vi "FormCalibra11-joao.vi"() -> ()   [LabVIEW 2014]
uses:
  testMachine.ctl
  mainMachine.ctl
  <vilib>/Instr/_visa.llb/VISA Configure Serial Port (Instr).vi
  <vilib>/express/express shared/transition.llb/Dynamic To Waveform Array.vi
  <vilib>/express/express signal manip/GetorSetDDTAttributes/Set DDT Attributes/SetT0.vi
  <vilib>/express/express shared/transition.llb/Waveform Array To Dynamic.vi
  <vilib>/express/express signal manip/GetorSetDDTAttributes/Set DDT Attributes/Set DDT Properties.xnode
panel:
  out "editVibration":dbl caption="Vibration (mg)" format="%#_4f"
  in  "editOffsetForce 3":dbl caption="Tare (Kgf)" min=-100.0 max=100.0 step=0.1
  out "editForce 3":dbl caption="Force (Kgf)" format="%#_4f"
  in  "editOffsetForce 2":dbl caption="Tare (Kgf)" min=-100.0 max=100.0 step=0.1
  out "editForce 2":dbl caption="Force (Kgf)" format="%#_4f"
  in  "editSetTempRefB":dbl caption="Offset B" step=0.01 format="%#_2f"
  in  "VISA Serial Port":refnum<visa-resource-name>
  in  "Lower level":dbl
  in  "hysteresis":dbl format="%.2p"
  in  "level":dbl format="%.2p"
  out "rpm":bool
  out "editTotalWaitLimit":u8
  out "editCountWaitLimit":u8
  out "ledWaitState":bool caption="Wait State"
  out "sliderWaitUpperTime":u8(slide) max=50 scale=0.0..30.0
  out "slideWaitLowerTime":u8(slide) max=30 scale=0.0..1.0
  out "slideWaitTime":u8(slide) scale=0.0..50.0
  out "labelTestTime":string caption="Tempo total de ensaio"
  in  "editSetWaitTime":u8 caption="Interval between snubs (s)" step=1 format="%0d"
  in  "stop":bool
  out "ledAcquireState":bool caption="Acquire State"
  out "editTotalLowerLimit":u8
  out "editCountLowerLimit":u8
  out "editTotalUpperLimit":u8
  out "editCountUpperLimit":u8
  out "ledEnsaio 3":bool
  out "ledBrakeState":bool caption="Brake State"
  out "ledExitState":bool caption="Exit State"
  out "ledMotorState":bool caption="Motor State"
  out "ledInit2State":bool caption="Init State"
  out "ledBlockState":bool caption="Block State"
  out "ledRunningState":bool caption="Running State"
  out "ledReadyState":bool caption="Ready State"
  out "ledInitState":bool caption="Init State"
  out "mainMachine":T1
  out "testMachine":T2=enum."finish"
  in  "editSetPathToFile":path
  in  "buttonStop":bool
  in  "buttonStart":bool
  in  "editOffsetForce":dbl caption="Tare (Kgf)" min=-100.0 max=100.0 step=0.1
  out "editForce":dbl caption="Force (Kgf)" format="%#_4f"
  out "editRPM":dbl caption="RPM" format="%#_4f"
  out "editFrequency":dbl caption="Frequency (Hz)" format="%#_4f"
  in  "editSetWaitLowerTime":u8 caption="Lower Wait Interval (s)"
  in  "editSetWaitUpperTime":u8=3 caption="Upper Wait Interval (s)"
  in  "editSetNumberOfCycles":u16 caption="Number of snubs" max=999 step=1 format="%0d"
  in  "editSetLowerLimit":u32 caption="Lower Limit (RPM)"
  in  "editSetUpperLimit":u32 caption="Upper Limit (RPM)"
  out "editTempB":dbl caption="Temperature B (ºC)"
  out "editTempA":dbl caption="Temperature A (ºC)"
  in  "editSetTempRefA":dbl caption="Offset A" step=0.01 format="%#_2f"
  out "ledMotor":bool
  out "ledBrake":bool
  out "ledEnsaio":bool
  out "labelTotalCycle":string
  out "labelCurrentCycle":string
  out "labelSystemTitle":string
  in  "editCurrCycleCtr":u32
  in  "velocidade 2":u32
  out "velocidade":u32
  # "Brake Test Bench"
  # "Com Port"
  # "Temperature"
  # "Rotation"
  # "Load Cell"
  # "Accelerometer"
  # "Test Configuration"
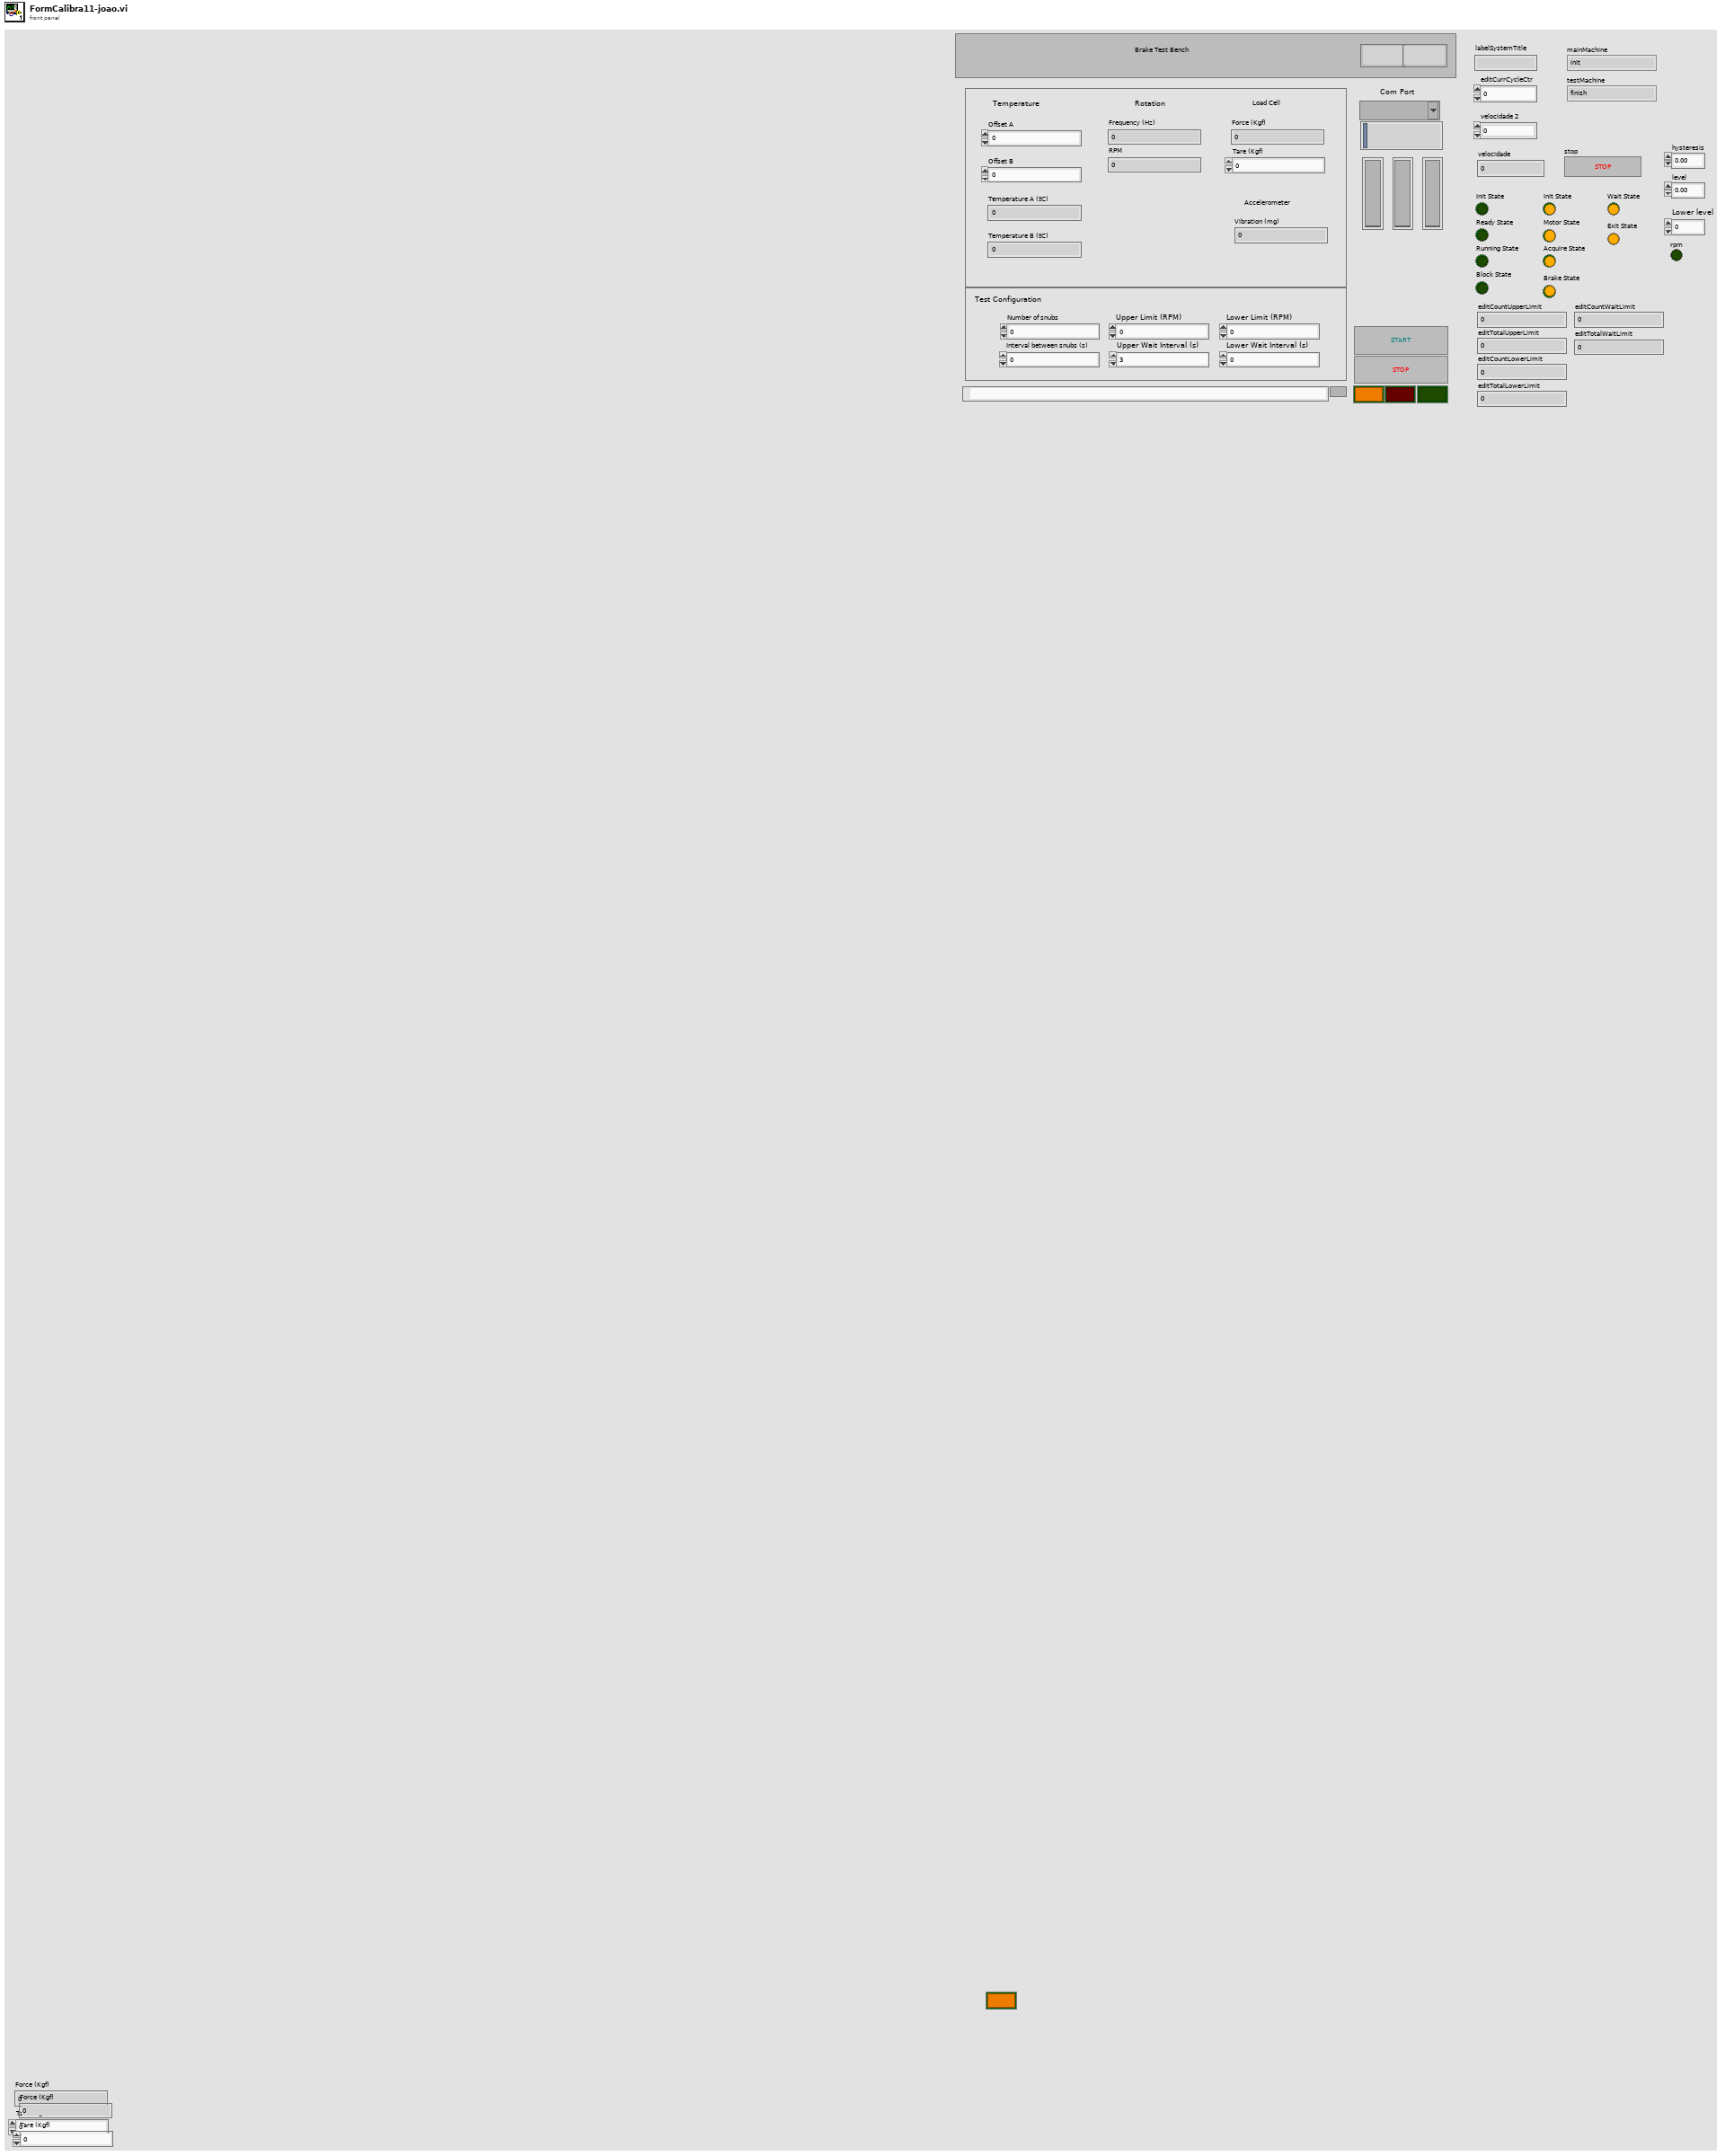
[diagram p1: front panel]
types:
  T1 = typedef "mainMachine.ctl" = enum16{"init", "ready", "running", "blocked", "finish"}
  T2 = typedef "testMachine.ctl" = enum16{"init", "motor", "motor acquire", "brake", "brake acquire", "wait ", "finish", "exit"}
  T3 = enum8{"Enabled", "Disabled", "Disabled and Grayed Out"}
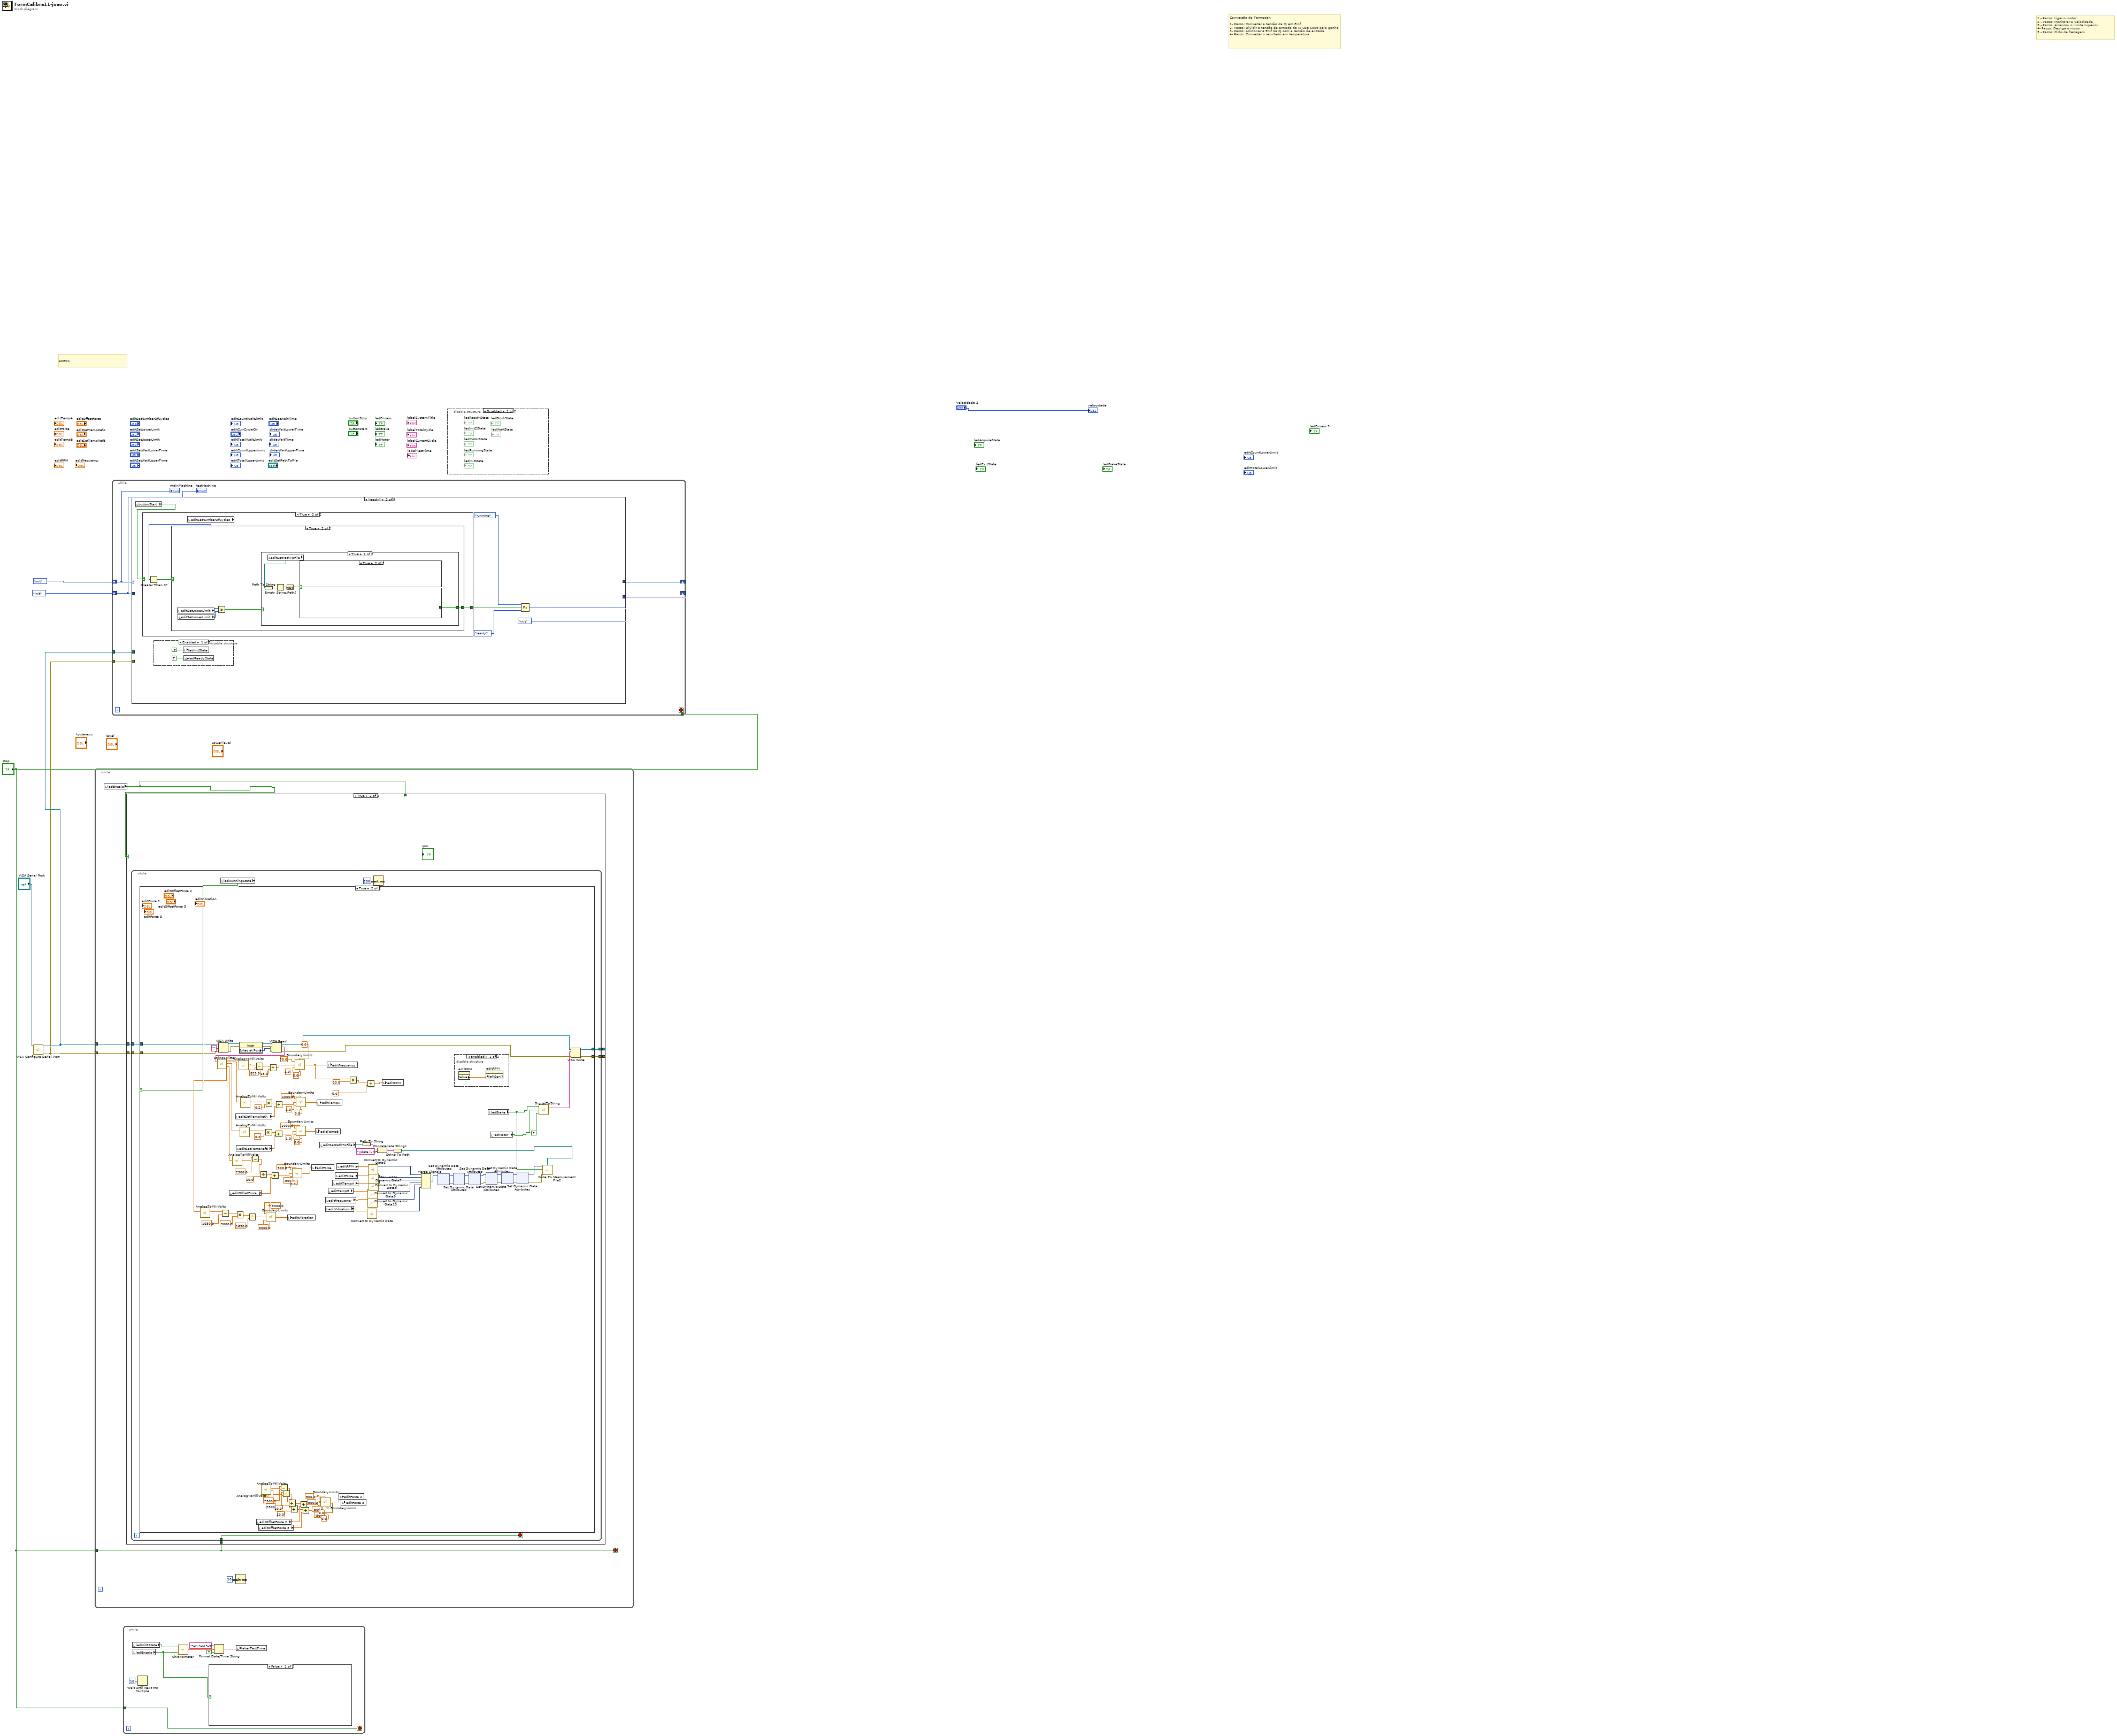
[diagram p0: block diagram]
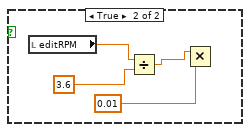
[diagram p3: hidden frame]
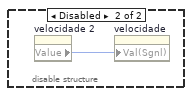
[diagram p6: hidden frame]
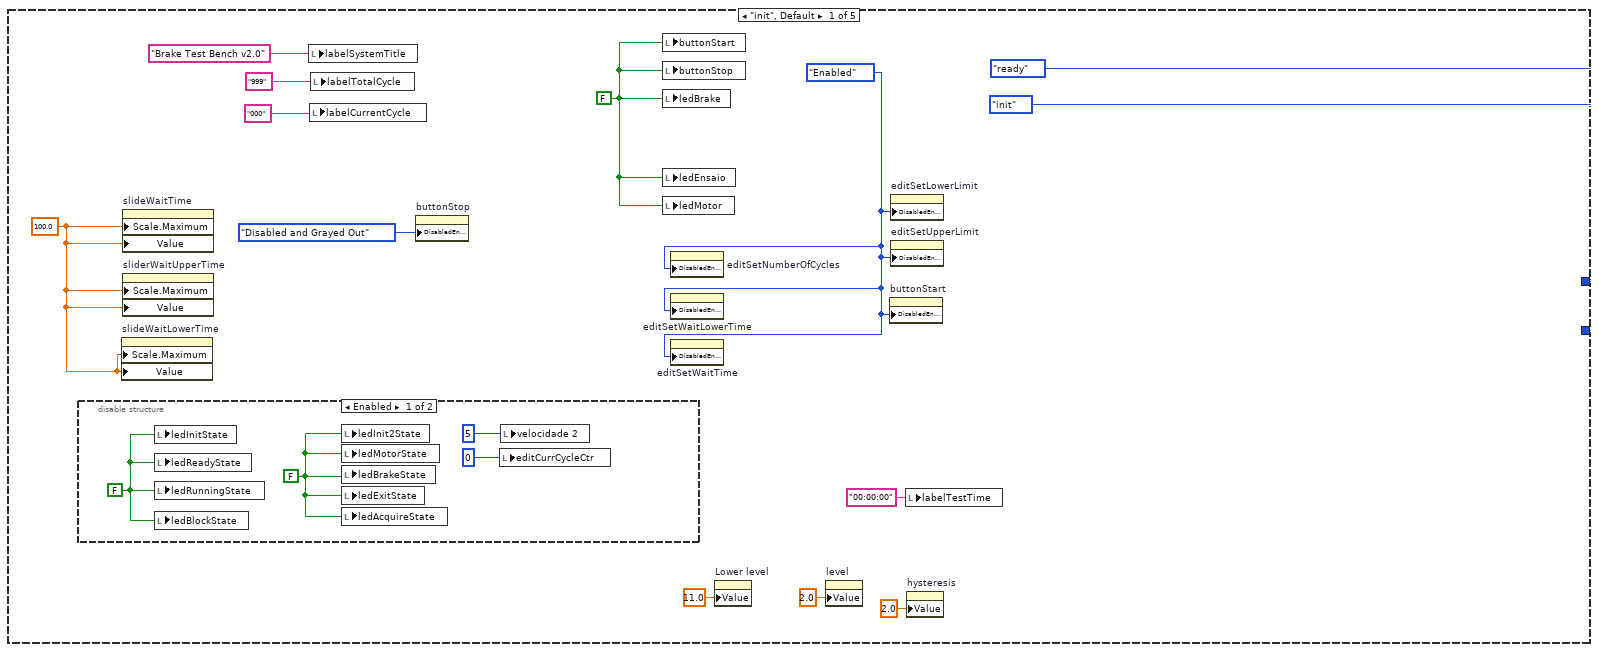
[diagram p7: hidden frame]
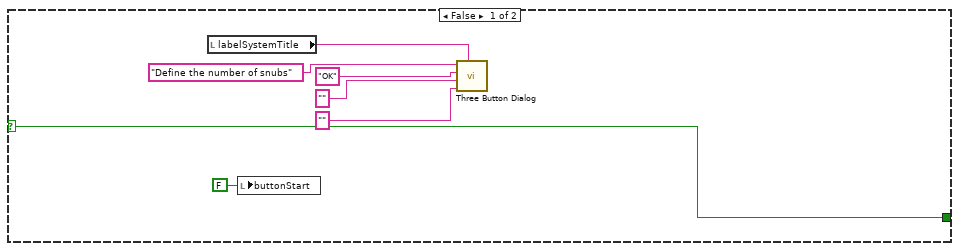
[diagram p11: hidden frame]
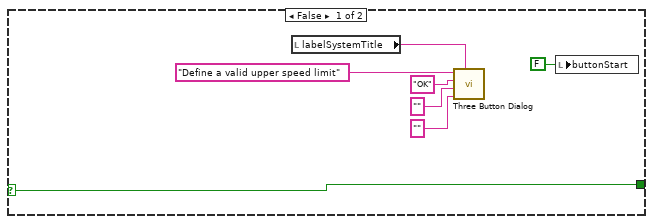
[diagram p12: hidden frame]
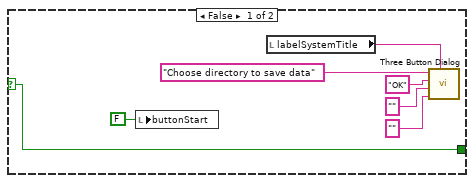
[diagram p13: hidden frame]
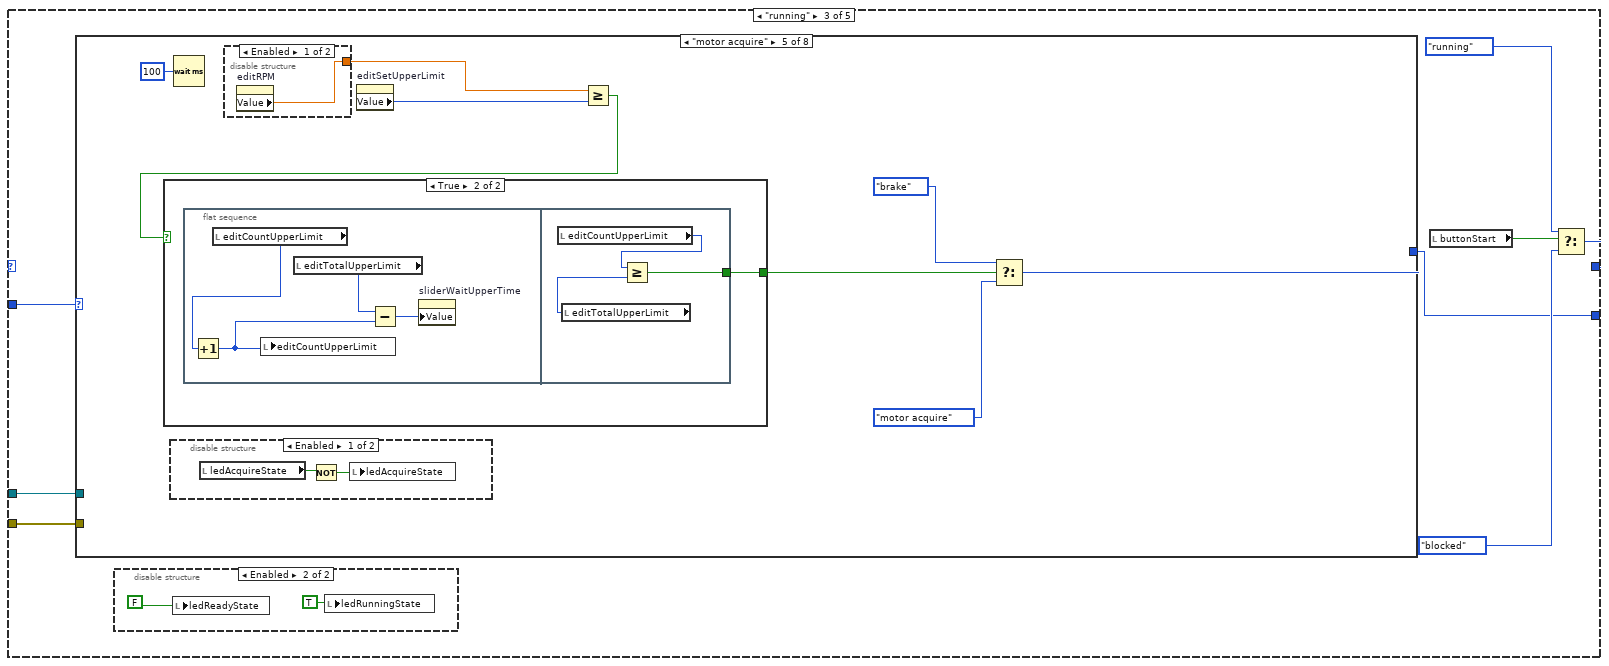
[diagram p14: hidden frame]
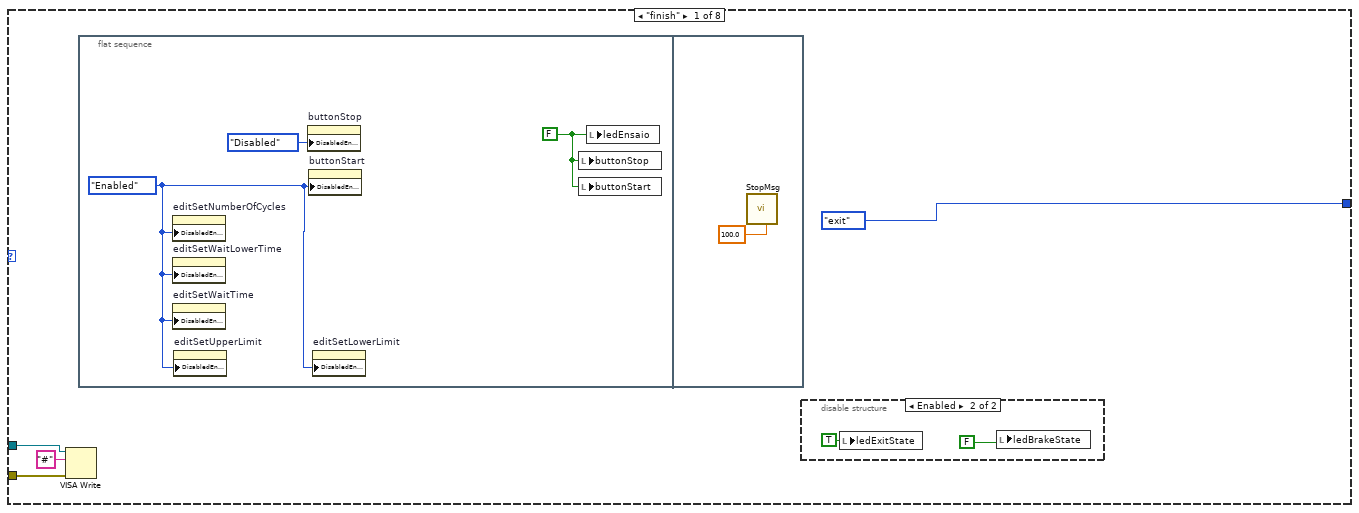
[diagram p16: hidden frame]
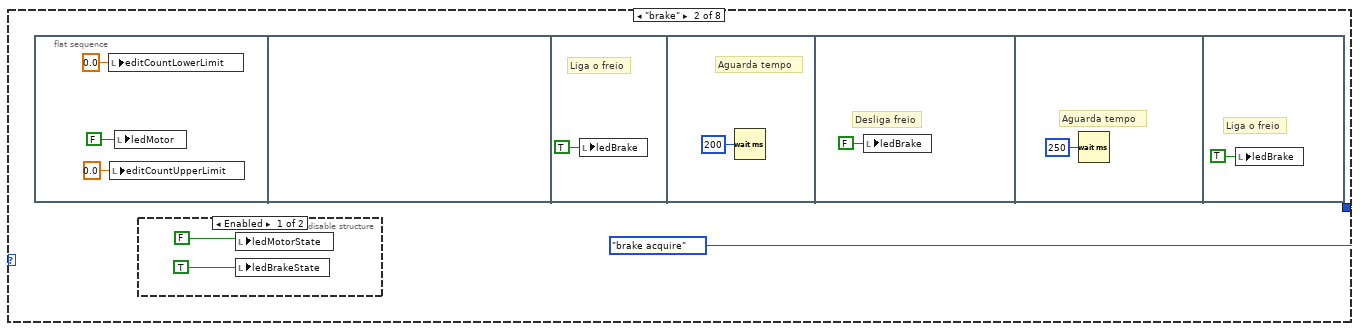
[diagram p18: hidden frame]
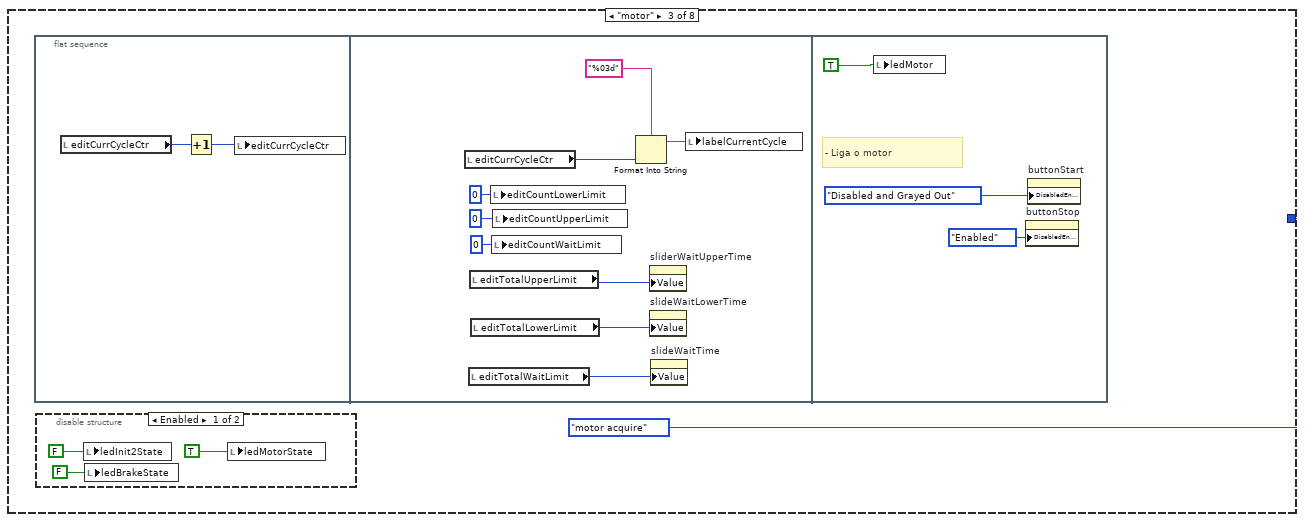
[diagram p20: hidden frame]
diagram:
  # "eSEDs"
  # "1 - Passo: Ligar o motor\n2 - Passo: Monitorar a velocidade\n3 - Passo: Alcancou o limite superior\n4- Passo: Desliga o motor\n5 - Passo: Ciclo de frenagem"
  # "Conversão do Termopar:\n\n1- Passo: Converter a tensão da CJ em Emf\n2- Passo: Dividir a tensão de entrada da NI USB 6009 pelo ganho\n3- Passo: Adicionar a Emf da CJ com a tensão de entrada\n4- Passo: Converter o resultado em temperatura"
  n1 = call-poly "VISA Configure Serial Port"("VISA resource name"="VISA Serial Port") -> ("VISA resource name out"=w3:refnum<visa-resource-name>, "error out"=w2:errorcluster)  [unwired: 13 in]
  n2 = while {
    tunnel: "stop" -> [w12]
    tunnel: w3 -> [w10]
    tunnel: w2 -> [w9]
    stop <- w12 stop-if-true
    n3 = local read "ledEnsaio"() -> (w8:bool)
    n4 = case shown="True" w8 {
      tunnel: w12 -> [_ w15]
      tunnel: w8 -> [_ _]
      tunnel: w10 -> [w14 w19]
      tunnel: w9 -> [w13 w18]
      tunnel: [w14 w17] -> _
      tunnel: [w13 w16] -> _
      frame False {
      }
      frame True {
        n5 = while {
          tunnel: w19 -> [w26]
          tunnel: w18 -> [w25]
          tunnel: [w24] -> w17
          tunnel: [w23] -> w16
          tunnel: w15 -> [w22]
          stop <- w22 stop-if-true
          n6 = local read "ledRunningState"() -> (w20:bool)
          n7 = case shown="True" w20 {
            tunnel: w26 -> [w28 w137]
            tunnel: w25 -> [w27 w136]
            tunnel: [w28 w133] -> w24
            tunnel: [w27 w132] -> w23
            frame False {
            }
            frame True {
              w36 = 3000.0
              w37 = 3000.0
              w56 = 500.0
              w67 = 500.0
              w109 = 500.0
              w126 = 1000.0
              w151 = 1000.0
              n8 = VISA Write(VISA resource name=w137, write buffer="!", error in (no error)=w136) -> (VISA resource name out=w141:refnum<visa-resource-name>, error out=w140:errorcluster)  [unwired: 1 out]
              n9 = local read "editOffsetForce"() -> (w105:dbl)
              n10 = local read "editSetTempRefA"() -> (w129:dbl)
              n11 = local read "editSetTempRefB"() -> (w120:dbl)
              n12 = property class="Instr"(reference=w141, error in=w140) -> (reference out=w144:refnum<visa-resource-name>, error out=w143:errorcluster, "Bytes at Port"=w142:u32)
              n13 = local read "editOffsetForce 2"() -> (w63:dbl)
              n14 = local read "editOffsetForce 3"() -> (w52:dbl)
              n15 = call "AnalogToMiliVolts.vi"() -> ("Output"=w60:dbl)  [unwired: 11 in]
              n16 = call "AnalogToMiliVolts.vi"() -> ("Output"=w49:dbl)  [unwired: 11 in]
              n17 = VISA Read(VISA resource name=w144, byte count=w142, error in (no error)=w143) -> (VISA resource name out=w135:refnum<visa-resource-name>, read buffer=w138:string, error out=w134:errorcluster)  [unwired: 1 out]
              n18 = call "StringSplitter.vi"("Input String"=w138) -> ("S0"=w155:dbl, "S1"=w145:dbl, "S2"=w118:dbl, "S4"=w98:dbl, "S5"=w43:dbl)  [unwired: 11 in, 3 out]
              n19 = call "AnalogToMiliVolts.vi"("Input"=w43) -> ("Output"=w45:dbl)  [unwired: 10 in]
              n20 = Subtract(x=w45, y=1650.0) -> (x-y=w42:dbl)
              n21 = call "AnalogToMiliVolts.vi"("Input"=w98) -> ("Output"=w100:dbl)  [unwired: 10 in]
              n22 = Multiply(x=w42, y=3000.0) -> (x*y=w40:dbl)
              n23 = call "AnalogToMiliVolts.vi"("Input"=w155) -> ("Output"=w110:dbl)  [unwired: 10 in]
              n24 = call "AnalogToMiliVolts.vi"("Input"=w118) -> ("Output"=w122:dbl)  [unwired: 10 in]
              n25 = call "AnalogToMiliVolts.vi"("Input"=w145) -> ("Output"=w146:dbl)  [unwired: 10 in]
              n26 = Divide(x=w40, y=1650.0) -> (x/y=w38:dbl)
              n27 = Subtract(x=w100, y=2500.0) -> (x-y=w99:dbl)
              n28 = Subtract(x=w110, y=825.0) -> (x-y=w117:dbl)
              n29 = Divide(x=w99, y=10.0) -> (x/y=w104:dbl)
              n30 = Multiply(x=w122, y=0.2) -> (x*y=w123:dbl)
              n31 = Multiply(x=w146, y=0.2) -> (x*y=w147:dbl)
              n32 = call "BoundaryLimits.vi"("UpperLimit"=w37, "UpperValue"=w37, "Input"=w38, "LowerLimit"=w36, "LowerValue"=w36) -> ("Output"=w35:dbl)
              n33 = Divide(x=w117, y=15.0) -> (x/y=w114:dbl)
              n34 = Add(x=w104, y=w105) -> (x+y=w106:dbl)
              n35 = Add(x=w123, y=w120) -> (x+y=w124:dbl)
              n36 = Add(x=w147, y=w129) -> (x+y=w148:dbl)
              n37 = Subtract(x=w60, y=2500.0) -> (x-y=w59:dbl)
              n38 = Subtract(x=w49, y=2500.0) -> (x-y=w48:dbl)
              n39 = local write "editVibration"(w35) -> ()
              n40 = Divide(x=w59, y=10.0) -> (x/y=w62:dbl)
              n41 = Divide(x=w48, y=10.0) -> (x/y=w51:dbl)
              n42 = call "BoundaryLimits.vi"("UpperLimit"=w109, "UpperValue"=w109, "Input"=w106, "LowerLimit"=-500.0, "LowerValue"=0.0) -> ("Output"=w102:dbl)
              n43 = call "BoundaryLimits.vi"("UpperLimit"=70.0, "UpperValue"=0.0, "Input"=w114, "LowerLimit"=1.0, "LowerValue"=0.0) -> ("Output"=w113:dbl)
              n44 = call "BoundaryLimits.vi"("UpperLimit"=w126, "UpperValue"=w126, "Input"=w124, "LowerLimit"=1.0, "LowerValue"=0.0) -> ("Output"=w119:dbl)
              n45 = call "BoundaryLimits.vi"("UpperLimit"=w151, "UpperValue"=w151, "Input"=w148, "LowerLimit"=1.0, "LowerValue"=0.0) -> ("Output"=w127:dbl)
              n46 = Add(x=w62, y=w63) -> (x+y=w64:dbl)
              n47 = Add(x=w51, y=w52) -> (x+y=w53:dbl)
              n48 = local write "editForce"(w102) -> ()
              n49 = local write "editTempB"(w119) -> ()
              n50 = local write "editTempA"(w127) -> ()
              n51 = local read "editSetPathToFile"() -> (w87:path)
              n52 = call "BoundaryLimits.vi"("UpperLimit"=w67, "UpperValue"=w67, "Input"=w64, "LowerLimit"=-500.0, "LowerValue"=0.0) -> ("Output"=w61:dbl)
              n53 = call "BoundaryLimits.vi"("UpperLimit"=w56, "UpperValue"=w56, "Input"=w53, "LowerLimit"=-500.0, "LowerValue"=0.0) -> ("Output"=w50:dbl)
              n54 = local read "editFrequency"() -> (w89:dbl)
              n55 = local read "editVibration"() -> (w34:dbl)
              n56 = local write "editFrequency"(w113) -> ()
              n57 = local read "editTempB"() -> (w90:dbl)
              n58 = local read "editTempA"() -> (w92:dbl)
              n59 = local read "editForce"() -> (w91:dbl)
              n60 = local read "editRPM"() -> (w77:dbl)
              n61 = local write "editForce 2"(w61) -> ()
              n62 = local write "editForce 3"(w50) -> ()
              n63 = Multiply(x=w113, y=10.0) -> (x*y=w112:dbl)
              n64 = Path To String(path=w87) -> (string=w88:string)
              n65 = Add(x=w112, y=0.0) -> (x+y=w111:dbl)
              n66 = call "Convert to Dynamic Data"("Double"=w34) -> ("Dynamic Data Type"=w33:dynamicdata)  [unwired: 3 in]
              n67 = call "Convert to Dynamic Data9"("Double"=w90) -> ("Dynamic Data Type"=w73:dynamicdata)  [unwired: 3 in]
              n68 = call "Convert to Dynamic Data10"("Double"=w89) -> ("Dynamic Data Type"=w72:dynamicdata)  [unwired: 3 in]
              n69 = call "Convert to Dynamic Data6"("Double"=w77) -> ("Dynamic Data Type"=w76:dynamicdata)  [unwired: 3 in]
              n70 = call "Convert to Dynamic Data7"("Double"=w91) -> ("Dynamic Data Type"=w75:dynamicdata)  [unwired: 3 in]
              n71 = call "Convert to Dynamic Data8"("Double"=w92) -> ("Dynamic Data Type"=w74:dynamicdata)  [unwired: 3 in]
              n72 = Concatenate Strings(w88, "\\data.lvm" ("string")) -> (w85:string)
              n73 = local write "editRPM"(w111) -> ()
              n74 = String To Path(string=w85) -> (path=w84:path)
              n75 = Merge Signals(w76, w75, w74, w73, w72, w33) -> (w68:dynamicdata)
              n76 = xnode ("Set Dynamic Data Attributes")("Signals In"=w68) -> ("Signals Out"=w83:dynamicdata, "error out"=w81:errorcluster)  [unwired: 4 in]
              n77 = xnode ("Set Dynamic Data Attributes")("Signals In"=w83, "error in"=w81) -> ("Signals Out"=w82:dynamicdata, "error out"=w80:errorcluster)  [unwired: 3 in]
              n78 = disable-structure shown="Enabled" {
                frame Enabled {
                  n79 = property on="editRPM" class="DigNum (strict)"() -> ("Value"=w264:dbl)  [unwired: 2 in, 2 out]
                  n80 = property on="editRPM" class="DigNum (strict)"("Val(Sgnl)"=w264) -> ()  [unwired: 2 in, 2 out]
                }
                frame Disabled {
                  n81 = property on="velocidade 2" class="DigNum (strict)"() -> ("Value"=w265:u32)  [unwired: 2 in, 2 out]
                  n82 = property on="velocidade" class="DigNum (strict)"("Val(Sgnl)"=w265) -> ()  [unwired: 2 in, 2 out]
                }
              }
              n83 = xnode ("Set Dynamic Data Attributes")("Signals In"=w82, "error in"=w80) -> ("Signals Out"=w71:dynamicdata, "error out"=w79:errorcluster)  [unwired: 3 in]
              n84 = xnode ("Set Dynamic Data Attributes")("Signals In"=w71, "error in"=w79) -> ("Signals Out"=w70:dynamicdata, "error out"=w78:errorcluster)  [unwired: 3 in]
              n85 = local read "ledBrake"() -> (w69:bool)
              n86 = local read "ledMotor"() -> (w101:bool)
              n87 = xnode ("Set Dynamic Data Attributes")("Signals In"=w70, "error in"=w78) -> ("Signals Out"=w32:dynamicdata, "error out"=w31:errorcluster)  [unwired: 3 in]
              n88 = xnode ("Set Dynamic Data Attributes")("Signals In"=w32, "error in"=w31) -> ("Signals Out"=w29:dynamicdata, "error out"=w30:errorcluster)  [unwired: 3 in]
              n89 = call "DigitalToString.vi"("D3"=FALSE, "D2"=w101, "D1"=w69) -> ("String"=w131:string)  [unwired: 1 out]
              n90 = call "Write To Measurement File2"("Signals"=w29, "Enable"=w69, "error in (no error)"=w30, "Filename"=w84) -> ()  [unwired: 13 in, 3 out]
              n91 = VISA Write(VISA resource name=w135, write buffer=w131, error in (no error)=w134) -> (VISA resource name out=w133:refnum<visa-resource-name>, error out=w132:errorcluster)  [unwired: 1 out]
            }
          }
          n92 = Wait (ms)(milliseconds to wait=u32 200) -> ()  [unwired: 1 out]
        }
      }
    }
    n93 = Wait (ms)(milliseconds to wait=u32 10) -> ()  [unwired: 1 out]
  }
  n94 = while {
    shift-right: [w272] -> _
    shift-left: mainMachine."init" ("mainMachine") -> [w269]
    shift-right: [w271] -> _
    shift-left: testMachine."init" ("testMachine") -> [w270]
    tunnel: "stop" -> [w268]
    tunnel: w3 -> [w267]
    tunnel: w2 -> [w266]
    stop <- w268 stop-if-true
    n95 = case shown="\"ready\"" w269 {
      tunnel: [mainMachine."ready" ("mainMachine") w290 w337 w486 mainMachine."finish" ("mainMachine")] -> w272
      tunnel: [testMachine."init" ("testMachine") testMachine."init" ("testMachine") w336 testMachine."init" ("testMachine") testMachine."init" ("testMachine")] -> w271
      tunnel: w270 -> [_ _ w335 _ _]
      tunnel: w267 -> [_ _ w334 _ _]
      tunnel: w266 -> [_ _ w333 _ _]
      frame "init", Default {
        w277 = 100.0 ("Scale.Range:Maximum")
        w278 = T3."Enabled" ("Disabled")
        w284 = FALSE ("motor")
        n96 = disable-structure shown="Enabled" {
          frame Enabled {
            w286 = FALSE
            w287 = FALSE
            n97 = local write "ledInitState"(w287) -> ()
            n98 = local write "ledReadyState"(w287) -> ()
            n99 = local write "ledRunningState"(w287) -> ()
            n100 = local write "ledBlockState"(w287) -> ()
            n101 = local write "ledInit2State"(w286) -> ()
            n102 = local write "ledMotorState"(w286) -> ()
            n103 = local write "ledBrakeState"(w286) -> ()
            n104 = local write "ledExitState"(w286) -> ()
            n105 = local write "ledAcquireState"(w286) -> ()
            n106 = local write "editCurrCycleCtr"(u32 0 ("currentCycleCtr")) -> ()
            n107 = local write "velocidade 2"(u32 5 ("velocidade 2")) -> ()
          }
          frame Disabled {
          }
        }
        n108 = property on="slideWaitLowerTime" class="Slide (strict)"("Scale.Maximum"=w277, "Value"=w277) -> ()  [unwired: 2 in, 2 out]
        n109 = property on="slideWaitTime" class="Slide (strict)"("Scale.Maximum"=w277, "Value"=w277) -> ()  [unwired: 2 in, 2 out]
        n110 = property on="sliderWaitUpperTime" class="Slide (strict)"("Scale.Maximum"=w277, "Value"=w277) -> ()  [unwired: 2 in, 2 out]
        n111 = local write "labelSystemTitle"("Brake Test Bench v2.0" ("systemTitle")) -> ()
        n112 = local write "labelCurrentCycle"("000" ("currentCycle")) -> ()
        n113 = local write "labelTotalCycle"("999" ("totalCycle")) -> ()
        n114 = property on="buttonStop" class="Bool (strict)"("DisabledEnum"=T3."Disabled and Grayed Out" ("Disabled")) -> ()  [unwired: 2 in, 2 out]
        n115 = local write "buttonStart"(w284) -> ()
        n116 = local write "buttonStop"(w284) -> ()
        n117 = local write "ledBrake"(w284) -> ()
        n118 = local write "ledEnsaio"(w284) -> ()
        n119 = local write "ledMotor"(w284) -> ()
        n120 = property on="editSetNumberOfCycles" class="DigNum (strict)"("DisabledEnum"=w278) -> ()  [unwired: 2 in, 2 out]
        n121 = property on="editSetWaitLowerTime" class="DigNum (strict)"("DisabledEnum"=w278) -> ()  [unwired: 2 in, 2 out]
        n122 = property on="editSetWaitTime" class="DigNum (strict)"("DisabledEnum"=w278) -> ()  [unwired: 2 in, 2 out]
        n123 = property on="Lower level" class="DigNum (strict)"("Value"=11.0 ("Lower level")) -> ()  [unwired: 2 in, 2 out]
        n124 = property on="level" class="DigNum (strict)"("Value"=2.0 ("level")) -> ()  [unwired: 2 in, 2 out]
        n125 = property on="buttonStart" class="Bool (strict)"("DisabledEnum"=w278) -> ()  [unwired: 2 in, 2 out]
        n126 = property on="editSetLowerLimit" class="DigNum (strict)"("DisabledEnum"=w278) -> ()  [unwired: 2 in, 2 out]
        n127 = property on="editSetUpperLimit" class="DigNum (strict)"("DisabledEnum"=w278) -> ()  [unwired: 2 in, 2 out]
        n128 = local write "labelTestTime"("00:00:00" ("labelTestTime")) -> ()
        n129 = property on="hysteresis" class="DigNum (strict)"("Value"=2.0 ("hysteresis")) -> ()  [unwired: 2 in, 2 out]
      }
      frame "ready" {
        n130 = local read "buttonStart"() -> (w293:bool)
        n131 = case shown="True" w293 {
          selector: w293 -> [w298 _]
          tunnel: [w298 w299] -> w292
          frame False {
          }
          frame True {
            n132 = local read "editSetNumberOfCycles"() -> (w300:u16)
            n133 = Greater Than 0?(x=w300) -> (x > 0?=w301:bool)
            n134 = case shown="True" w301 {
              selector: w301 -> [w308 _]
              tunnel: [w308 w309] -> w299
              frame False {
                n135 = local read "labelSystemTitle"() -> (w303:string)
                n136 = local write "buttonStart"(FALSE ("startButton")) -> ()
                n137 = call <vilib>:"Three Button Dialog.vi"("Window Title (\"\")"=w303, "Right Button Text (\"Cancel\")"="" ("Right Button Text (\"Cancel\")"), "Center Button Text (\"No\")"="" ("Center Button Text (\"No\")"), "Left Button Text (\"Yes\")"="OK" ("Left Button Text (\"Yes\")"), "message"="Define the number of snubs") -> ()  [unwired: 6 in, 1 out]
              }
              frame True {
                n138 = local read "editSetUpperLimit"() -> (w311:u32)
                n139 = local read "editSetLowerLimit"() -> (w310:u32)
                n140 = Greater?(x=w311, y=w310) -> (0:w312:bool)
                n141 = case shown="True" w312 {
                  selector: w312 -> [w319 _]
                  tunnel: [w319 w322] -> w309
                  frame False {
                    n142 = local read "labelSystemTitle"() -> (w314:string)
                    n143 = call <vilib>:"Three Button Dialog.vi"("Window Title (\"\")"=w314, "Right Button Text (\"Cancel\")"="" ("Right Button Text (\"Cancel\")"), "Center Button Text (\"No\")"="" ("Center Button Text (\"No\")"), "Left Button Text (\"Yes\")"="OK" ("Left Button Text (\"Yes\")"), "message"="Define a valid upper speed limit") -> ()  [unwired: 6 in, 1 out]
                    n144 = local write "buttonStart"(FALSE ("startButton")) -> ()
                  }
                  frame True {
                    n145 = local read "editSetPathToFile"() -> (w324:path)
                    n146 = Path To String(path=w324) -> (string=w323:string)
                    n147 = Empty String/Path?(string/path=w323) -> (empty?=w321:bool)
                    n148 = Not(x=w321) -> (.not. x?=w320:bool)
                    n149 = case shown="True" w320 {
                      selector: w320 -> [w331 w332]
                      tunnel: [w331 w332] -> w322
                      frame False {
                        n150 = local write "buttonStart"(FALSE ("startButton")) -> ()
                        n151 = local read "labelSystemTitle"() -> (w326:string)
                        n152 = call <vilib>:"Three Button Dialog.vi"("Window Title (\"\")"=w326, "Right Button Text (\"Cancel\")"="" ("Right Button Text (\"Cancel\")"), "Center Button Text (\"No\")"="" ("Center Button Text (\"No\")"), "Left Button Text (\"Yes\")"="OK" ("Left Button Text (\"Yes\")"), "message"="Choose directory to save data") -> ()  [unwired: 6 in, 1 out]
                      }
                      frame True {
                      }
                    }
                  }
                }
              }
            }
          }
        }
        n153 = disable-structure shown="Enabled" {
          frame Enabled {
            n154 = local write "ledInitState"(FALSE ("ledReady")) -> ()
            n155 = local write "ledReadyState"(TRUE ("ledReady")) -> ()
          }
          frame Disabled {
          }
        }
        n156 = Select(t=mainMachine."running" ("mainMachine"), s=w292, f=mainMachine."ready" ("mainMachine")) -> (s? t:f=w290:T1)
      }
      frame "running" {
        n157 = case shown="\"motor acquire\"" w335 {
          tunnel: [testMachine."exit" ("testMachine") testMachine."brake acquire" ("testMachine") testMachine."motor acquire" ("testMachine") testMachine."motor" ("testMachine") w416 w436 testMachine."exit" ("testMachine") w469] -> w336
          tunnel: w334 -> [w344 _ _ w383 _ _ _ _]
          tunnel: w333 -> [w343 _ _ w382 _ _ _ _]
          frame "finish" {
            n158 = VISA Write(VISA resource name=w344, write buffer="#", error in (no error)=w343) -> ()  [unwired: 3 out]
            n159 = flat-sequence {
              frame #0 {
                w350 = FALSE ("ledReady")
                w349 = T3."Enabled" ("Disabled")
                n160 = property on="editSetNumberOfCycles" class="DigNum (strict)"("DisabledEnum"=w349) -> ()  [unwired: 2 in, 2 out]
                n161 = property on="editSetWaitLowerTime" class="DigNum (strict)"("DisabledEnum"=w349) -> ()  [unwired: 2 in, 2 out]
                n162 = property on="editSetWaitTime" class="DigNum (strict)"("DisabledEnum"=w349) -> ()  [unwired: 2 in, 2 out]
                n163 = property on="editSetUpperLimit" class="DigNum (strict)"("DisabledEnum"=w349) -> ()  [unwired: 2 in, 2 out]
                n164 = property on="buttonStop" class="Bool (strict)"("DisabledEnum"=T3."Disabled" ("Disabled")) -> ()  [unwired: 2 in, 2 out]
                n165 = property on="buttonStart" class="Bool (strict)"("DisabledEnum"=w349) -> ()  [unwired: 2 in, 2 out]
                n166 = property on="editSetLowerLimit" class="DigNum (strict)"("DisabledEnum"=w349) -> ()  [unwired: 2 in, 2 out]
                n167 = local write "buttonStop"(w350) -> ()
                n168 = local write "buttonStart"(w350) -> ()
                n169 = local write "ledEnsaio"(w350) -> ()
              }
              frame #1 {
                n170 = call "StopMsg.vi"("Max Value (100)"=100.0) -> ()  [unwired: 8 in, 2 out]
              }
            }
            n171 = disable-structure shown="Enabled" {
              frame Disabled {
              }
              frame Enabled {
                n172 = local write "ledExitState"(TRUE ("ledReady")) -> ()
                n173 = local write "ledBrakeState"(FALSE ("ledReady")) -> ()
              }
            }
          }
          frame "brake" {
            n174 = flat-sequence {
              frame #0 {
                n175 = local write "editCountLowerLimit"(0.0 ("editCountUpperLimit")) -> ()
                n176 = local write "editCountUpperLimit"(0.0 ("editCountUpperLimit")) -> ()
                n177 = local write "ledMotor"(FALSE ("motor")) -> ()
              }
              frame #1 {
              }
              frame #2 {
                # "Liga o freio"
                n178 = local write "ledBrake"(TRUE ("freio")) -> ()
              }
              frame #3 {
                # "Aguarda tempo"
                n179 = Wait (ms)(milliseconds to wait=u32 200) -> ()  [unwired: 1 out]
              }
              frame #4 {
                # "Desliga freio"
                n180 = local write "ledBrake"(FALSE ("freio")) -> ()
              }
              frame #5 {
                # "Aguarda tempo"
                n181 = Wait (ms)(milliseconds to wait=u32 250) -> ()  [unwired: 1 out]
              }
              frame #6 {
                # "Liga o freio"
                n182 = local write "ledBrake"(TRUE ("freio")) -> ()
              }
            }
            n183 = disable-structure shown="Enabled" {
              frame Enabled {
                n184 = local write "ledMotorState"(FALSE ("ledReady")) -> ()
                n185 = local write "ledBrakeState"(TRUE ("ledReady")) -> ()
              }
              frame Disabled {
              }
            }
          }
          frame "motor" {
            n186 = flat-sequence {
              frame #0 {
                n187 = local read "editCurrCycleCtr"() -> (w369:u32)
                n188 = Increment(x=w369) -> (x+1=w368:u32)
                n189 = local write "editCurrCycleCtr"(w368) -> ()
              }
              frame #1 {
                n190 = local read "editCurrCycleCtr"() -> (w376:u32)
                n191 = local read "editTotalWaitLimit"() -> (w370:u8)
                n192 = local read "editTotalUpperLimit"() -> (w372:u8)
                n193 = local read "editTotalLowerLimit"() -> (w371:u8)
                n194 = local write "editCountLowerLimit"(u8 0 ("editCountLowerLimit")) -> ()
                n195 = local write "editCountWaitLimit"(u8 0 ("editCountWaitLimit")) -> ()
                n196 = local write "editCountUpperLimit"(u8 0 ("editCountUpperLimit")) -> ()
                n197 = Format Into String(format string="%03d", w376) -> (resulting string=w377:string)  [unwired: 2 in, 1 out]
                n198 = property on="sliderWaitUpperTime" class="Slide (strict)"("Value"=w372) -> ()  [unwired: 2 in, 2 out]
                n199 = property on="slideWaitLowerTime" class="Slide (strict)"("Value"=w371) -> ()  [unwired: 2 in, 2 out]
                n200 = property on="slideWaitTime" class="Slide (strict)"("Value"=w370) -> ()  [unwired: 2 in, 2 out]
                n201 = local write "labelCurrentCycle"(w377) -> ()
              }
              frame #2 {
                # "- Liga o motor"
                n202 = local write "ledMotor"(TRUE ("motor")) -> ()
                n203 = property on="buttonStop" class="Bool (strict)"("DisabledEnum"=T3."Enabled" ("Disabled")) -> ()  [unwired: 2 in, 2 out]
                n204 = property on="buttonStart" class="Bool (strict)"("DisabledEnum"=T3."Disabled and Grayed Out" ("Disabled")) -> ()  [unwired: 2 in, 2 out]
              }
            }
            n205 = disable-structure shown="Enabled" {
              frame Enabled {
                n206 = local write "ledInit2State"(FALSE ("ledReady")) -> ()
                n207 = local write "ledBrakeState"(FALSE ("ledReady")) -> ()
                n208 = local write "ledMotorState"(TRUE ("ledReady")) -> ()
              }
              frame Disabled {
              }
            }
          }
          frame "init", Default {
            n209 = stacked-sequence {
              tunnel: w383 -> [_ _ _]
              tunnel: w382 -> [_ _ _]
              frame #0 {
                w391 = FALSE ("ensaio")
                n210 = local write "ledMotor"(w391) -> ()
                n211 = local write "ledBrake"(w391) -> ()
                n212 = local read "editSetNumberOfCycles"() -> (w398:u16)
                n213 = local read "editSetWaitLowerTime"() -> (w392:u8)
                n214 = local read "editSetWaitUpperTime"() -> (w395:u8)
                n215 = local read "editSetWaitTime"() -> (w386:u8)
                n216 = Multiply(x=w386, y=u32 10) -> (x*y=w387:u32)
                n217 = Multiply(x=w392, y=u32 10) -> (x*y=w390:u32)
                n218 = Format Into String(format string="%03d", w398) -> (resulting string=w399:string)  [unwired: 2 in, 1 out]
                n219 = Multiply(x=w395, y=u32 10) -> (x*y=w389:u32)
                n220 = local write "editTotalLowerLimit"(w390) -> ()
                n221 = local write "editTotalUpperLimit"(w389) -> ()
                n222 = local write "editTotalWaitLimit"(w387) -> ()
                n223 = local write "labelTotalCycle"(w399) -> ()
                n224 = local write "editCurrCycleCtr"(u32 0 ("currentCycleCtr")) -> ()
                n225 = local write "labelCurrentCycle"("000" ("currentCycle")) -> ()
              }
              frame #1 {
                w407 = T3."Disabled" ("Disabled")
                n226 = property on="editSetNumberOfCycles" class="DigNum (strict)"("DisabledEnum"=w407) -> ()  [unwired: 2 in, 2 out]
                n227 = property on="editSetWaitLowerTime" class="DigNum (strict)"("DisabledEnum"=w407) -> ()  [unwired: 2 in, 2 out]
                n228 = property on="editSetWaitTime" class="DigNum (strict)"("DisabledEnum"=w407) -> ()  [unwired: 2 in, 2 out]
                n229 = local read "editTotalUpperLimit"() -> (w410:u8)
                n230 = property on="sliderWaitUpperTime" class="Slide (strict)"("Scale.Maximum"=w410, "Scale.Minimum"=0.0 ("Scale.Range:Minimum"), "Scale.Increment"=1.0 ("Scale.Range:Increment"), "Value"=w410) -> ()  [unwired: 2 in, 2 out]
                n231 = local read "editTotalLowerLimit"() -> (w404:u8)
                n232 = property on="slideWaitLowerTime" class="Slide (strict)"("Scale.Maximum"=w404, "Scale.Minimum"=0.0 ("Scale.Range:Minimum"), "Scale.Increment"=1.0 ("Scale.Range:Increment"), "Value"=w404) -> ()  [unwired: 2 in, 2 out]
                n233 = local read "editTotalWaitLimit"() -> (w401:u8)
                n234 = property on="slideWaitTime" class="Slide (strict)"("Scale.Maximum"=w401, "Scale.Minimum"=0.0 ("Scale.Range:Minimum"), "Scale.Increment"=1.0 ("Scale.Range:Increment"), "Value"=w401) -> ()  [unwired: 2 in, 2 out]
                n235 = call "StarMsg.vi"("Show"=TRUE, "Max Value (100)"=100.0) -> ()  [unwired: 7 in, 2 out]
                n236 = property on="editSetLowerLimit" class="DigNum (strict)"("DisabledEnum"=w407) -> ()  [unwired: 2 in, 2 out]
                n237 = property on="editSetUpperLimit" class="DigNum (strict)"("DisabledEnum"=w407) -> ()  [unwired: 2 in, 2 out]
              }
              frame #2 {
                n238 = local write "ledEnsaio"(TRUE ("ensaio")) -> ()
              }
            }
            n239 = disable-structure shown="Enabled" {
              frame Enabled {
                n240 = local write "ledInit2State"(TRUE ("ledReady")) -> ()
              }
              frame Disabled {
              }
            }
          }
          frame "motor acquire" {
            n241 = disable-structure shown="Enabled" {
              frame Enabled {
                n242 = local read "ledAcquireState"() -> (w425:bool)
                n243 = Not(x=w425) -> (.not. x?=w424:bool)
                n244 = local write "ledAcquireState"(w424) -> ()
              }
              frame Disabled {
              }
            }
            n245 = Wait (ms)(milliseconds to wait=u32 100) -> ()  [unwired: 1 out]
            n246 = disable-structure shown="Enabled" {
              disable-tunnel: [w422 w423] -> w415
              frame Enabled {
                n247 = property on="editRPM" class="DigNum (strict)"() -> ("Value"=w422:dbl)  [unwired: 2 in, 2 out]
              }
              frame Disabled {
                n248 = property on="velocidade" class="DigNum (strict)"() -> ("Value"=w423:u32)  [unwired: 2 in, 2 out]
              }
            }
            n249 = property on="editSetUpperLimit" class="DigNum (strict)"() -> ("Value"=w414:u32)  [unwired: 2 in, 2 out]
            n250 = Greater Or Equal?(x=w415, y=w414) -> (x >= y?=w420:bool)
            n251 = case shown="True" w420 {
              selector: w420 -> [w426 _]
              tunnel: [w426 w427] -> w419
              frame False {
              }
              frame True {
                n252 = flat-sequence {
                  tunnel: [w432] -> w427
                  frame #0 {
                    n253 = local read "editCountUpperLimit"() -> (w430:u8)
                    n254 = Increment(x=w430) -> (x+1=w428:u8)
                    n255 = local write "editCountUpperLimit"(w428) -> ()
                    n256 = local read "editTotalUpperLimit"() -> (w429:u8)
                    n257 = Subtract(x=w429, y=w428) -> (x-y=w431:u8)
                    n258 = property on="sliderWaitUpperTime" class="Slide (strict)"("Value"=w431) -> ()  [unwired: 2 in, 2 out]
                  }
                  frame #1 {
                    n259 = local read "editCountUpperLimit"() -> (w434:u8)
                    n260 = local read "editTotalUpperLimit"() -> (w433:u8)
                    n261 = Greater Or Equal?(x=w434, y=w433) -> (x >= y?=w432:bool)
                  }
                }
              }
            }
            n262 = Select(t=testMachine."brake" ("testMachine"), s=w419, f=testMachine."motor acquire" ("testMachine")) -> (s? t:f=w416:T2)
          }
          frame "brake acquire" {
            n263 = disable-structure shown="Enabled" {
              frame Enabled {
                n264 = local read "ledAcquireState"() -> (w444:bool)
                n265 = Not(x=w444) -> (.not. x?=w443:bool)
                n266 = local write "ledAcquireState"(w443) -> ()
              }
              frame Disabled {
              }
            }
            n267 = Wait (ms)(milliseconds to wait=u32 100) -> ()  [unwired: 1 out]
            n268 = disable-structure shown="Enabled" {
              disable-tunnel: [w445 w446] -> w435
              frame Enabled {
                n269 = property on="editRPM" class="DigNum (strict)"() -> ("Value"=w445:dbl)  [unwired: 2 in, 2 out]
              }
              frame Disabled {
                n270 = property on="velocidade" class="DigNum (strict)"() -> ("Value"=w446:u32)  [unwired: 2 in, 2 out]
              }
            }
            n271 = property on="editSetLowerLimit" class="DigNum (strict)"() -> ("Value"=w437:u32)  [unwired: 2 in, 2 out]
            n272 = Less Or Equal?(x=w435, y=w437) -> (x <= y?=w441:bool)
            n273 = case shown="True" w441 {
              selector: w441 -> [w447 _]
              tunnel: [w447 w448] -> w439
              frame False {
              }
              frame True {
                n274 = flat-sequence {
                  tunnel: [w454] -> w449
                  tunnel: w449 -> [w458]
                  tunnel: [w457] -> w448
                  frame #0 {
                    n275 = local read "editCountLowerLimit"() -> (w453:u8)
                    n276 = Increment(x=w453) -> (x+1=w452:u8)
                    n277 = local write "editCountLowerLimit"(w452) -> ()
                    n278 = local read "editTotalLowerLimit"() -> (w451:u8)
                    n279 = Subtract(x=w451, y=w452) -> (x-y=w450:u8)
                    n280 = property on="slideWaitLowerTime" class="Slide (strict)"("Value"=w450) -> ()  [unwired: 2 in, 2 out]
                  }
                  frame #1 {
                    n281 = local read "editCountLowerLimit"() -> (w456:u8)
                    n282 = local read "editTotalLowerLimit"() -> (w455:u8)
                    n283 = Greater Or Equal?(x=w456, y=w455) -> (x >= y?=w454:bool)
                  }
                  frame #2 {
                    n284 = case shown="True" w458 {
                      selector: w458 -> [w459 w460]
                      tunnel: [w459 w460] -> w457
                      frame False {
                      }
                      frame True {
                        # "- Desliga o freio"
                        n285 = local write "ledBrake"(FALSE ("freio")) -> ()
                      }
                    }
                  }
                }
              }
            }
            n286 = Select(t=testMachine."wait " ("testMachine"), s=w439, f=testMachine."brake acquire" ("testMachine")) -> (s? t:f=w436:T2)
          }
          frame "exit" {
          }
          frame "wait " {
            # "- Aguarda 0.5s \n- Atualiza o numero de ciclos"
            n287 = flat-sequence {
              tunnel: [w475] -> w463
              frame #0 {
                n288 = local read "editCountWaitLimit"() -> (w471:u8)
                n289 = Increment(x=w471) -> (x+1=w472:u8)
                n290 = local write "editCountWaitLimit"(w472) -> ()
                n291 = local read "editTotalWaitLimit"() -> (w474:u8)
                n292 = Subtract(x=w474, y=w472) -> (x-y=w473:u8)
                n293 = property on="slideWaitTime" class="Slide (strict)"("Value"=w473) -> ()  [unwired: 2 in, 2 out]
              }
              frame #1 {
                n294 = local read "editCountWaitLimit"() -> (w477:u8)
                n295 = local read "editTotalWaitLimit"() -> (w476:u8)
                n296 = Greater Or Equal?(x=w477, y=w476) -> (x >= y?=w475:bool)
              }
            }
            n297 = disable-structure shown="Enabled" {
              frame Enabled {
                n298 = local read "ledWaitState"() -> (w484:bool)
                n299 = Not(x=w484) -> (.not. x?=w483:bool)
                n300 = local write "ledBrakeState"(FALSE ("ledBrakeState")) -> ()
                n301 = local write "ledWaitState"(w483) -> ()
              }
              frame Disabled {
              }
            }
            n302 = Wait (ms)(milliseconds to wait=u32 100) -> ()  [unwired: 1 out]
            n303 = case shown="True" w463 {
              selector: w463 -> [w478 _]
              tunnel: [w478 w482] -> w464
              frame False {
              }
              frame True {
                n304 = local read "editSetNumberOfCycles"() -> (w480:u16)
                n305 = local read "editCurrCycleCtr"() -> (w479:u32)
                n306 = Greater Or Equal?(x=w479, y=w480) -> (x >= y?=w482:bool)
                n307 = Not(x=w482) -> (.not. x?=w481:bool)
                n308 = local write "ledEnsaio"(w481) -> ()
              }
            }
            n309 = Select(t=testMachine."motor" ("testMachine"), s=w463, f=testMachine."wait " ("testMachine")) -> (s? t:f=w465:T2)
            n310 = Select(t=testMachine."finish" ("testMachine"), s=w464, f=w465) -> (s? t:f=w469:T2)
          }
        }
        n311 = disable-structure shown="Enabled" {
          frame Disabled {
          }
          frame Enabled {
            n312 = local write "ledReadyState"(FALSE ("ledReady")) -> ()
            n313 = local write "ledRunningState"(TRUE ("ledReady")) -> ()
          }
        }
        n314 = local read "buttonStart"() -> (w340:bool)
        n315 = Select(t=mainMachine."running" ("mainMachine"), s=w340, f=mainMachine."blocked" ("mainMachine")) -> (s? t:f=w337:T1)
      }
      frame "blocked" {
        n316 = local read "buttonStart"() -> (w490:bool)
        n317 = Select(t=mainMachine."ready" ("mainMachine"), s=w490, f=mainMachine."blocked" ("mainMachine")) -> (s? t:f=w486:T1)
        n318 = local write "ledRunningState"(FALSE ("ledReady")) -> ()
        n319 = local write "ledBlockState"(TRUE ("ledReady")) -> ()
      }
      frame "finish" {
        n320 = local write "ledBlockState"(FALSE ("ledReady")) -> ()
      }
    }
    "mainMachine" <- w269
    "testMachine" <- w270
  }
  n321 = while {
    tunnel: "stop" -> [w503]
    stop <- w503 stop-if-true
    n322 = local read "ledInit2State"() -> (w498:bool)
    n323 = local read "ledEnsaio"() -> (w496:bool)
    n324 = Wait Until Next ms Multiple(millisecond multiple=u32 10) -> ()  [unwired: 1 out]
    n325 = call "Chronometer.vi"("start"=w496, "reset"=w498) -> ("Time"=w502:dbl)
    n326 = case shown="False" w496 {
      frame False {
      }
      frame True {
        n327 = local read "editRPM"() -> (w506:dbl)
        n328 = Divide(x=w506, y=3.6) -> (x/y=w504:dbl)
        n329 = Multiply(x=w504, y=0.01) -> ()  [unwired: 1 out]
      }
    }
    n330 = Format Date/Time String(time format string (%c)="%H:%M:%S", seconds (now)=w502, UTC format=TRUE) -> (date/time string=w499:string)
    n331 = local write "labelTestTime"(w499) -> ()
  }
  n332 = disable-structure shown="Disabled" {
    frame Disabled {
    }
    frame Enabled {
    }
  }
  "velocidade" <- "velocidade 2"
